vi "stopwatch_kernel.vi"(9 "State variables in":cluster{"Timestamp":dbl, "Elapsed Time":dbl}, 11 "Command":enum16{"Elapsed Time", "Reset"}(ring)) -> (1 "State variables out":cluster{"Timestamp":dbl, "Elapsed Time":dbl}, 3 "Elapsed Time":dbl)   [LabVIEW 2015]
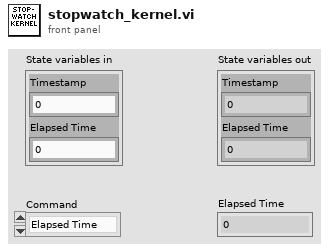
[diagram p1: front panel]
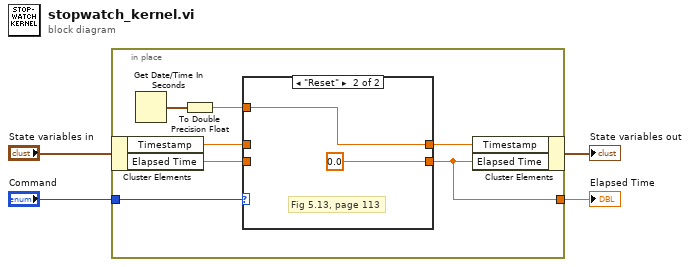
[diagram p0: block diagram]
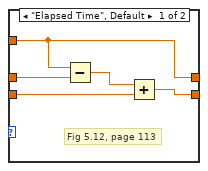
[diagram p2: hidden frame]
diagram:
  n1 = in-place {
    in-place-border: "Command" -> [w6]
    in-place-border: [w5] -> w1
    n2 = in-place-cluster #1("State variables in") -> ("Timestamp"=w9:dbl, "Elapsed Time"=w8:dbl)
    n3 = Get Date/Time In Seconds() -> (seconds since 1Jan1904=w11:timestamp)
    n4 = To Double Precision Float(number=w11) -> (double precision float=w10:dbl)
    n5 = case shown="\"Reset\"" w6 {
      tunnel: w10 -> [w12 w18]
      tunnel: w9 -> [w16 _]
      tunnel: w8 -> [w15 _]
      tunnel: [w12 w18] -> w7
      tunnel: [w13 0.0] -> w5
      frame "Elapsed Time", Default {
        # "Fig 5.12, page 113"
        n6 = Subtract(x=w12, y=w16) -> (x-y=w14:dbl)
        n7 = Add(x=w14, y=w15) -> (x+y=w13:dbl)
      }
      frame "Reset" {
        # "Fig 5.13, page 113"
      }
    }
    n8 = in-place-cluster #1("Timestamp"=w7, "Elapsed Time"=w5) -> (→"State variables out":cluster{"Timestamp":dbl, "Elapsed Time":dbl})
  }
  "Elapsed Time" <- w1
